vi "MegaAwesome_8_29_12a_JW.vi"() -> ()   [LabVIEW 2011]
uses:
  MegaAwesome_States.ctl
panel:
  out "Folder Index":dbl caption="Length"
  out "Image Preview":T1(plugin-control)
  out "Sat Id-Used":dbl[](array[numeric])
  out "Sat Vg Array-Used":dbl[](array[numeric])
  out "Vg Array-Log-Used":dbl[](array[numeric])
  out "Sat Id-Log-Used":dbl[](array[numeric])
  out "Lin Id-Used":dbl[](array[numeric])
  out "Lin-Vg Array-Used":dbl[](array[numeric])
  out "Lin Vd":dbl
  out "Recorded Prop":T2
  out "Current State":T3
  in  "Main Tab Control":T4(tab)
  in  "Image Folder":path
  out "Image File":path=path "D:/UserData/Desktop/Jeremy/WFU/Research/Programs/VI mods/Image Not Found.png"
  in  "Transfer File":path
  out "Transfer Folder":path
  out "Fabrication Prop":T5
  in  "File Controls":T6
  out "Date Recorded":string="Date Recorded" caption="Measured"
  out "Data Name:":string
  out "Image Name":string
  out "Index":string
  out "Date Created":string caption="Fabricated"
  in  "Comments:":string
  out "Rec: Length":dbl caption="Length" format="%#_3g"
  out "Rec: Width":dbl caption="Width" format="%#_4g"
  out "Rec: Dielectric (d)":dbl caption="Dielectric (d)" format="%#_3g"
  in  "New: Dielectric":dbl
  in  "New: Length":dbl
  in  "New: Width":dbl
  out "Rec: Temp":dbl caption="Sample Temp" format="%.1f"
  in  "New: Temp":dbl format="%.1f"
  in  "Independant Variable":string(combo)="Length (um):"
  out "Image Out":T1(plugin-control)
  in  "Num Pts":dbl=5.0
  in  "Num Pts Log":dbl=5.0 caption="Num Pts"
  out "Recorded Values Cluster":T7
  out "Calculated Values Cluster":T7 caption="Recorded Values Cluster"
  out "Re-Calculated Values Cluster":T7 caption="Recorded Values Cluster"
  in  "Origin Project File":path=path "\\\\acad1\\physics/Jurchescu-group/JW-PD/Group Library/Origin Project Files/DeviceData_8_10_12a_JW.opj"
  in  "No Image File":path=path "\\\\acad1\\physics/Jurchescu-group/JW-PD/Mega Awesome/Image Not Found.png"
  in  "Room Temp":dbl=294.0
  # "Image Location"
  # "Recorded"
  # "Calculated"
  # "Re-Calculated"
  # "Manual"
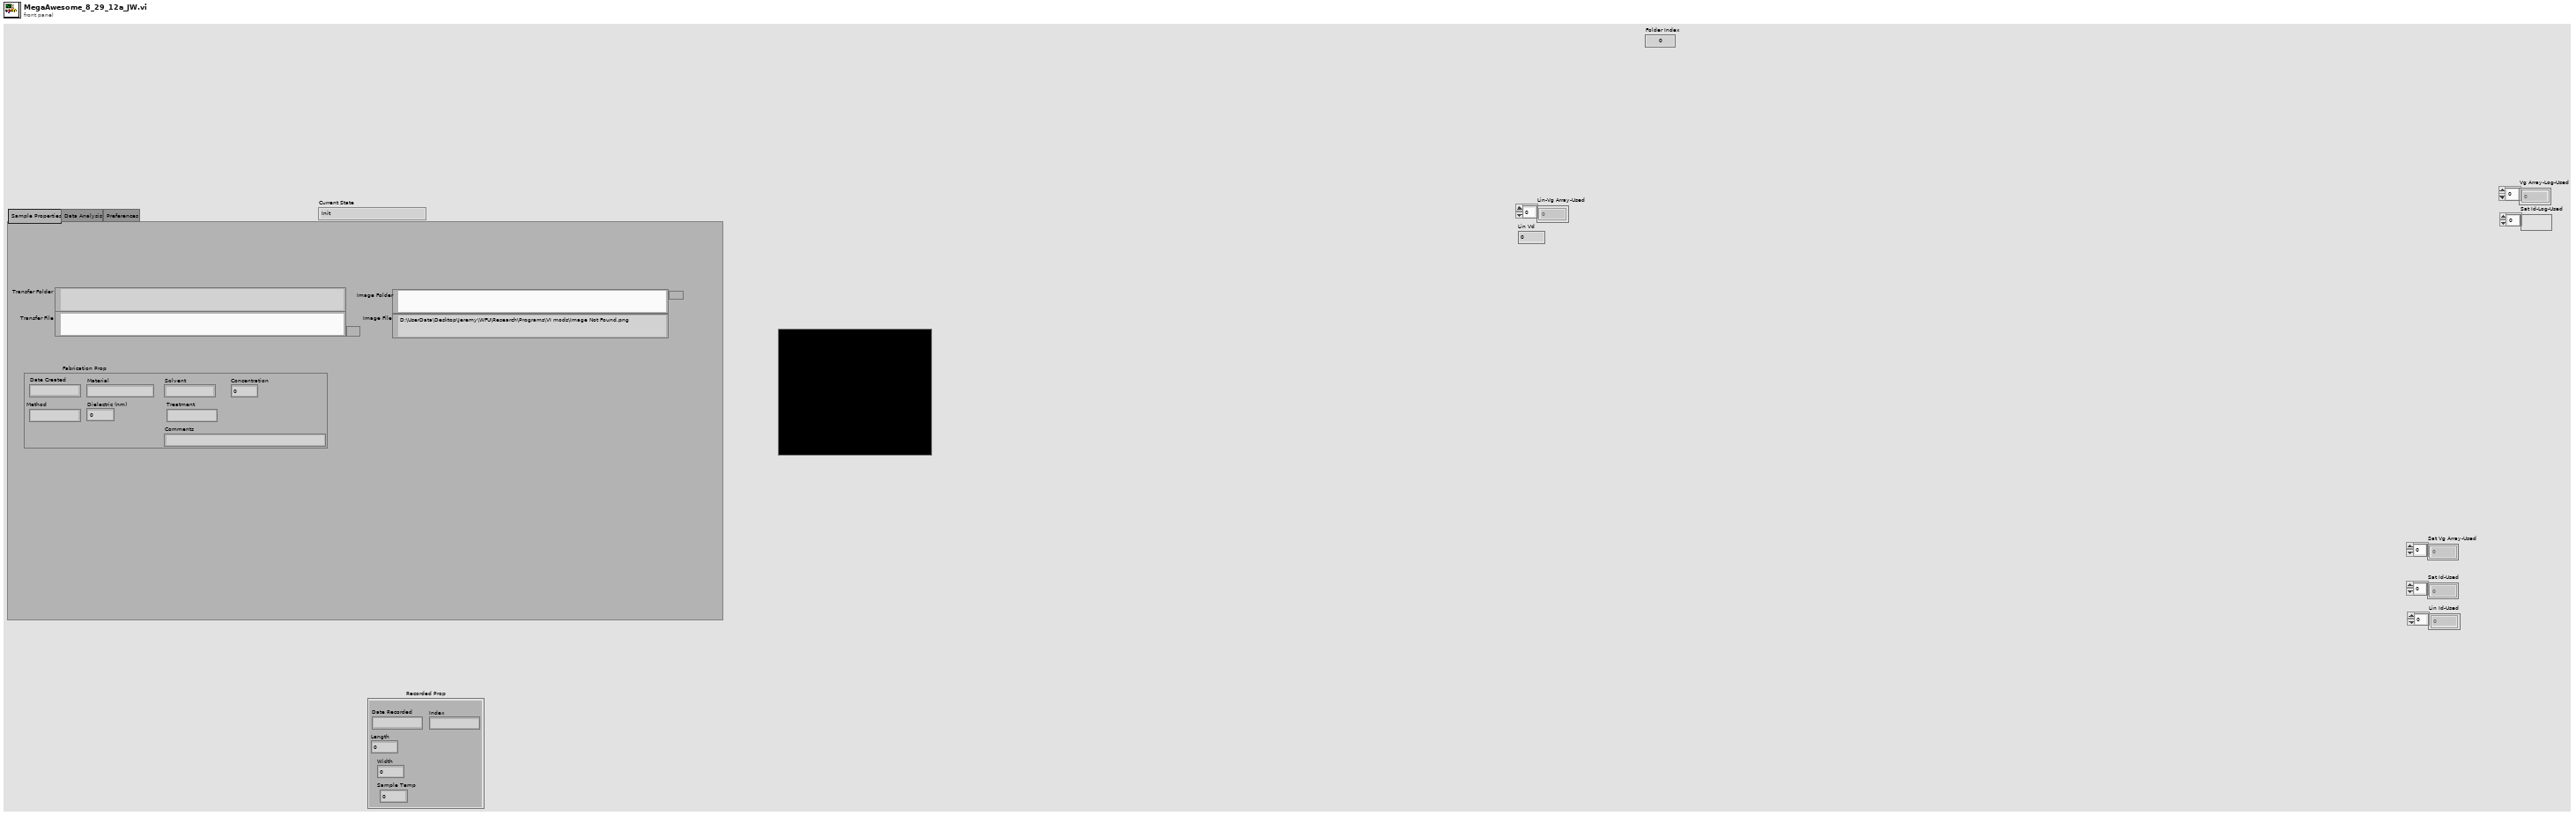
[diagram p1: front panel]
types:
  T1 = typedef "IMAQ Image.ctl" = refnum<image>
  T2 = cluster{"Date Recorded":string, "Index":string, "Length":dbl, "Width":dbl, "Sample Temp":dbl}
  T3 = typedef "MegaAwesome_States.ctl" = enum16{"Init", "File Missing", "No Event", "Read Data", "Calculated Values", "Re-Calculated Values", "Next File", "Previous File", "Discard File", "Save", "Save Lines", "Export", "Exit"}
  T4 = enum32{"Sample Properties", "Data Analysis", "Preferences"}
  T5 = cluster{"Date Created":string, "Material":string, "Solvent":string, "Concentration":dbl, "Method":string, "Dielectric (nm)":dbl, "Treatment":string, "Comments":string}
  T6 = cluster{"Previous File":bool, "Discard ":bool, "Save Lines":bool, "Close":bool, "Next File ":bool, "Save":bool, "Save Next":bool, "Export":bool}
  T7 = cluster{"Mobility-Sat":dbl, "Moblitity-Lin":dbl, "On/Off":dbl, "Off Current":dbl, "Vt-Sat":dbl, "STS":dbl, "Trap Density-VT":dbl, "Trap Density-STS":dbl}
  T8 = cluster{"Mobility-Sat":dbl, "Vt-Sat":dbl, "Mobility-Lin":dbl, "Vt-Lin":dbl, "Off I-Sat":dbl, "On/Off I-Sat":dbl}
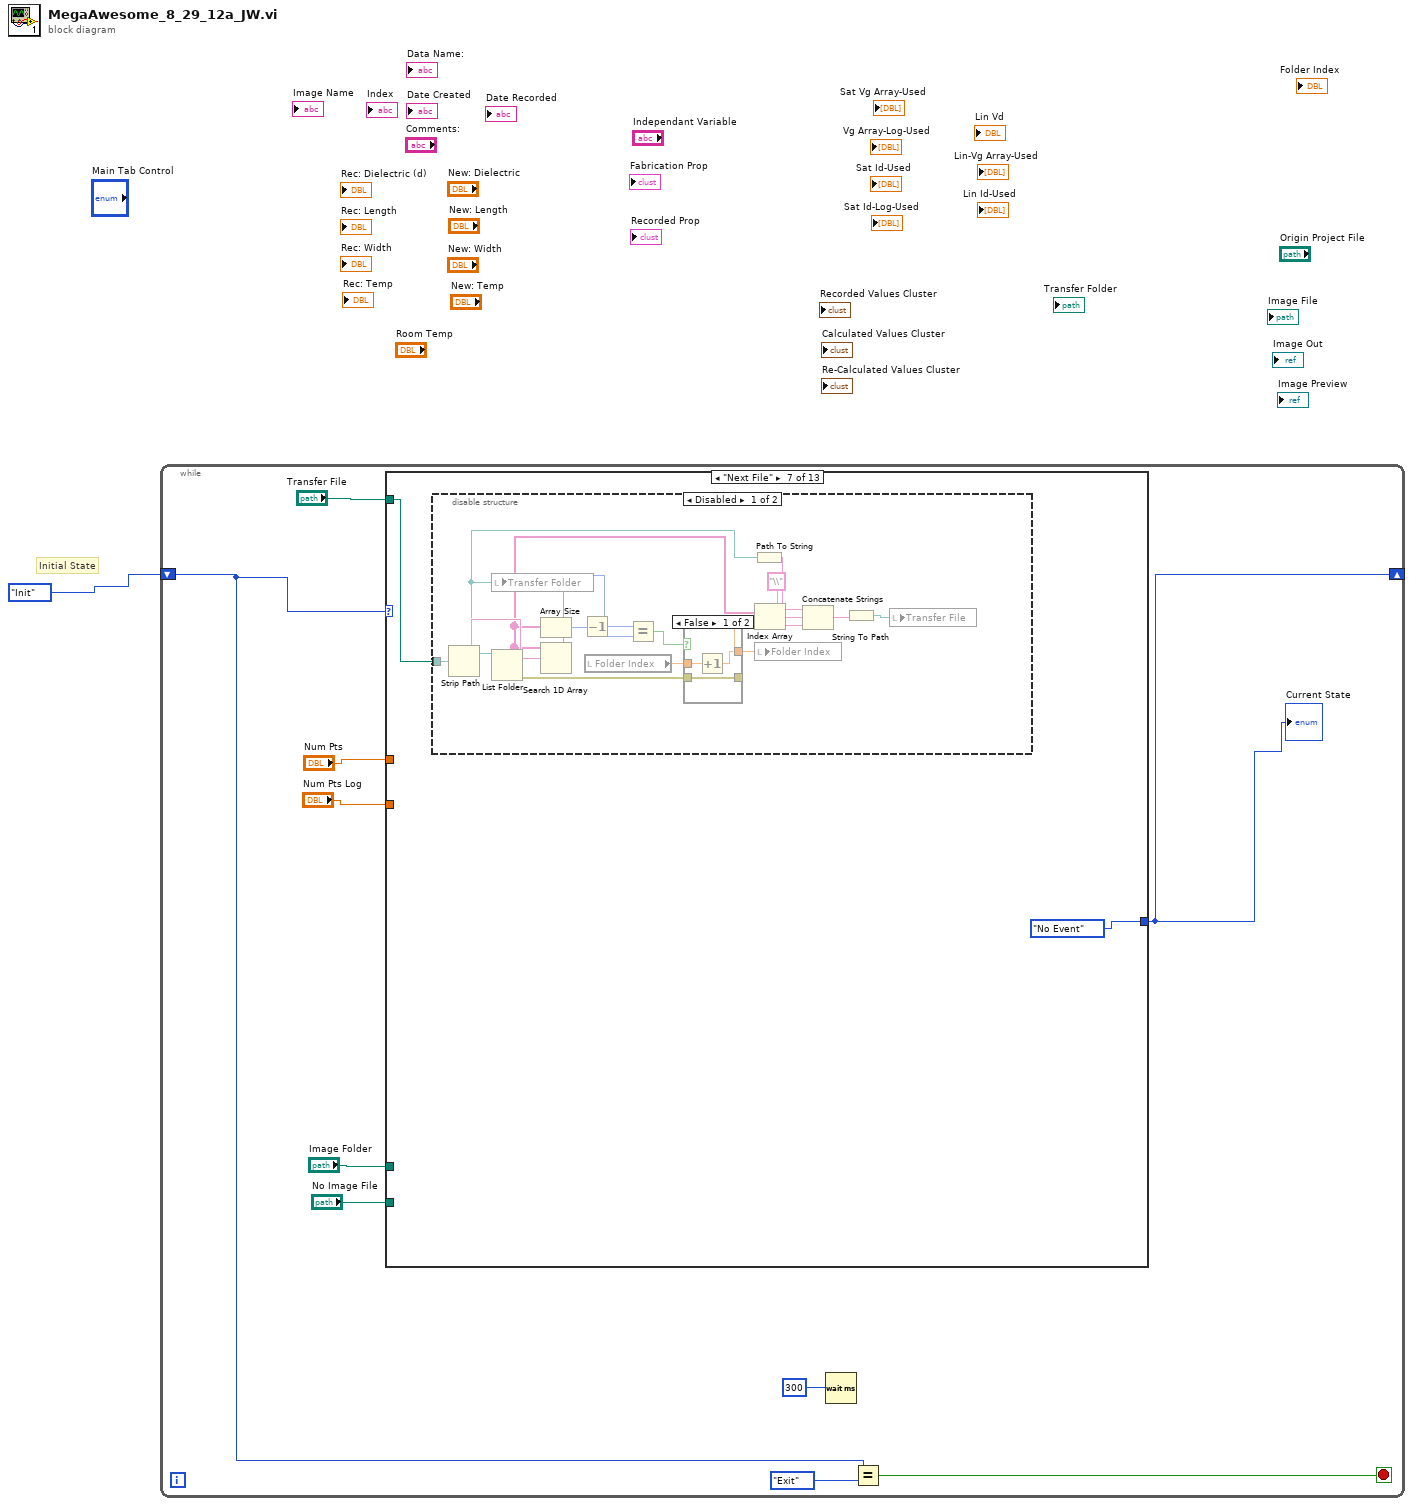
[diagram p0: block diagram]
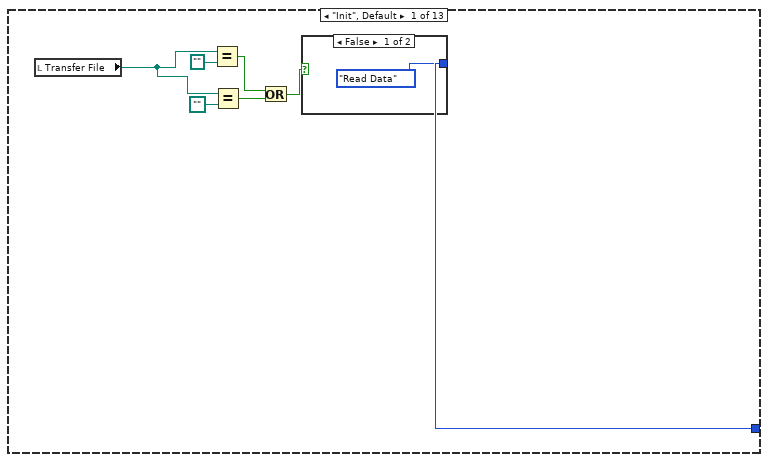
[diagram p2: hidden frame]
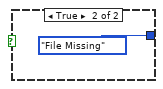
[diagram p3: hidden frame]
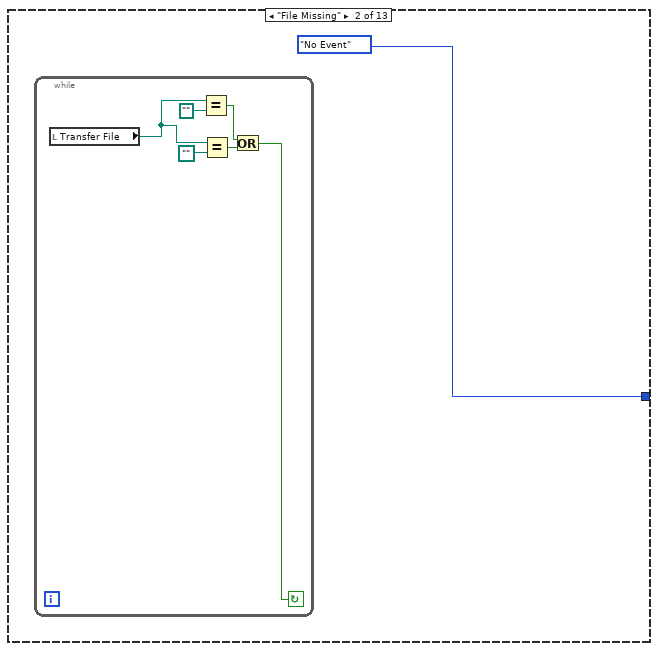
[diagram p4: hidden frame]
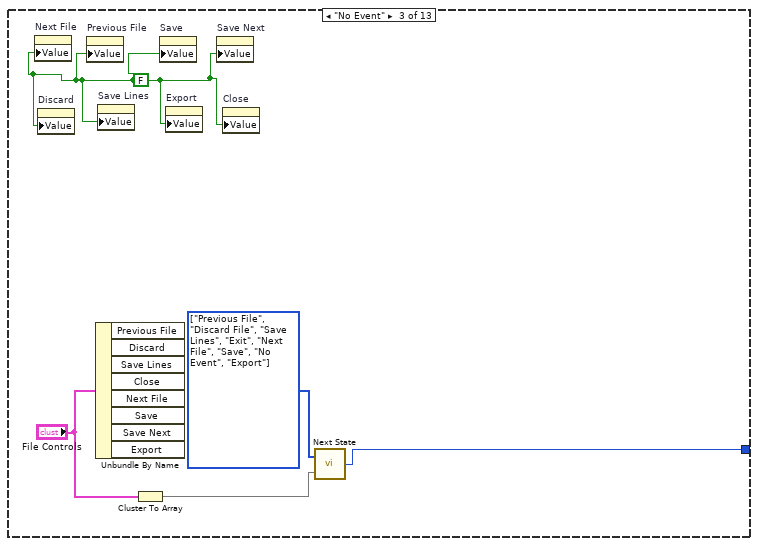
[diagram p5: hidden frame]
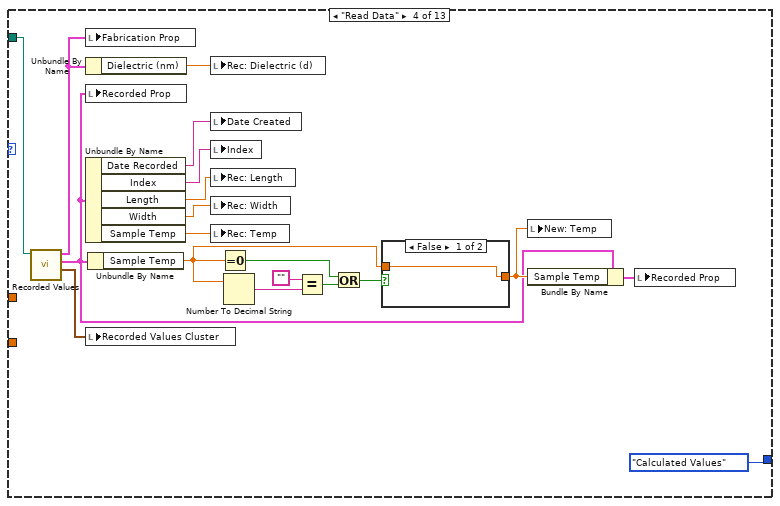
[diagram p6: hidden frame]
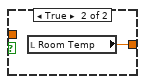
[diagram p7: hidden frame]
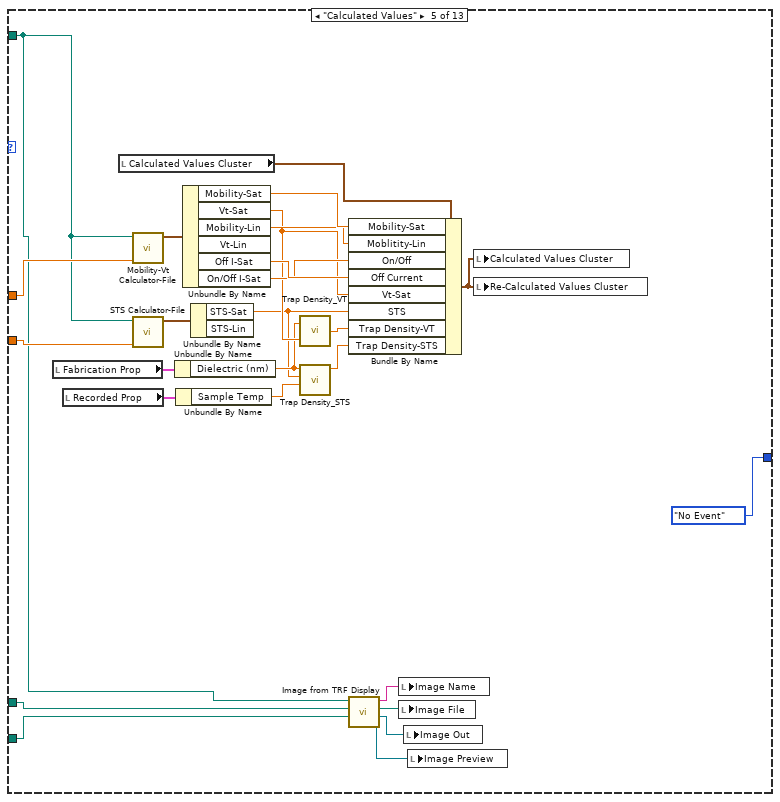
[diagram p8: hidden frame]
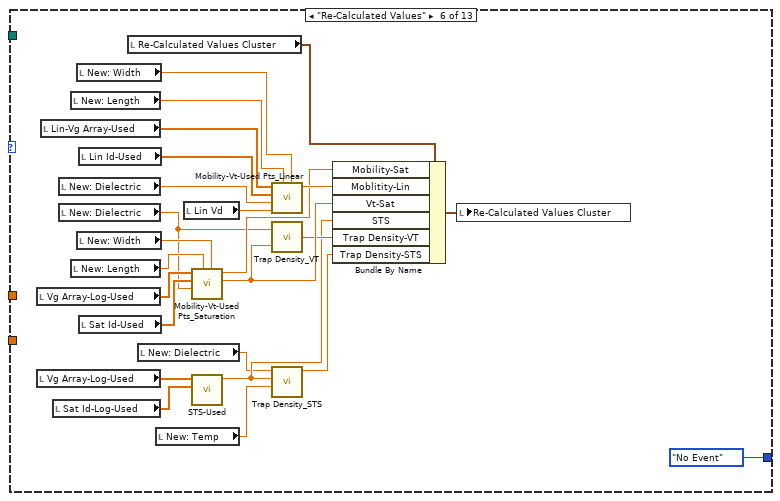
[diagram p9: hidden frame]
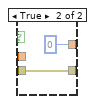
[diagram p10: hidden frame]
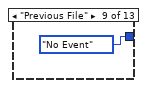
[diagram p13: hidden frame]
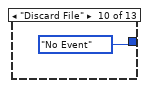
[diagram p14: hidden frame]
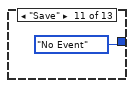
[diagram p15: hidden frame]
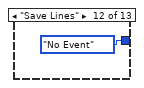
[diagram p16: hidden frame]
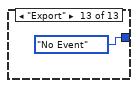
[diagram p17: hidden frame]
diagram:
  # "Initial State"
  n1 = while {
    shift-right: [w7] -> _
    shift-left: MegaAwesome_States."Init" -> [w10]
    stop <- w11 stop-if-true
    n2 = case shown="\"Next File\"" w10 {
      selector: w10 -> [_ _ _ _ _ _ _ w127 _ _ _ _ _]
      tunnel: [w12 MegaAwesome_States."No Event" w30 MegaAwesome_States."Calculated Values" MegaAwesome_States."No Event" MegaAwesome_States."No Event" MegaAwesome_States."No Event" w127 MegaAwesome_States."No Event" MegaAwesome_States."No Event" MegaAwesome_States."No Event" MegaAwesome_States."No Event" MegaAwesome_States."No Event"] -> w7
      tunnel: "Transfer File" -> [_ _ _ w51 w60 _ w105 _ _ _ _ _ _]
      tunnel: "Num Pts" -> [_ _ _ _ w64 _ _ _ _ _ _ _ _]
      tunnel: "Num Pts Log" -> [_ _ _ _ w63 _ _ _ _ _ _ _ _]
      tunnel: "Image Folder" -> [_ _ _ _ w59 _ _ _ _ _ _ _ _]
      tunnel: "No Image File" -> [_ _ _ _ w58 _ _ _ _ _ _ _ _]
      frame "Init", Default {
        n3 = local read "Transfer File"() -> (w13:path)
        n4 = Equal?(x=w13, y=path "") -> (x = y?=w16:bool)
        n5 = Equal?(x=w13, y=path "") -> (x = y?=w15:bool)
        n6 = Or(x=w16, y=w15) -> (x .or. y?=w18:bool)
        n7 = case shown="False" w18 {
          tunnel: [MegaAwesome_States."Read Data" MegaAwesome_States."File Missing"] -> w12
          frame False {
          }
          frame True {
          }
        }
      }
      frame "File Missing" {
        n8 = while {
          stop <- w22 continue-if-true
          n9 = local read "Transfer File"() -> (w23:path)
          n10 = Equal?(x=w23, y=path "") -> (x = y?=w25:bool)
          n11 = Equal?(x=w23, y=path "") -> (x = y?=w26:bool)
          n12 = Or(x=w25, y=w26) -> (x .or. y?=w22:bool)
        }
      }
      frame "No Event" {
        w31 = T3[] [enum."Previous File", enum."Discard File", enum."Save Lines", enum."Exit", enum."Next File", enum."Save", enum."No Event", enum."Export"] items=["Init", "File Missing", "No Event", "Read Data", "Calculated Values", "Re-Calculated Values", "Next File", "Previous File", "Discard File", "Save", "Save Lines", "Export", "Exit"]
        w32 = FALSE
        n13 = property on="Next File" class="Bool (strict)"("Value"=w32) -> ()  [unwired: 2 in, 2 out]
        n14 = property on="Discard" class="Bool (strict)"("Value"=w32) -> ()  [unwired: 2 in, 2 out]
        n15 = property on="Previous File" class="Bool (strict)"("Value"=w32) -> ()  [unwired: 2 in, 2 out]
        n16 = Unbundle By Name("File Controls") -> ()  [unwired: 8 out]
        n17 = property on="Save Lines" class="Bool (strict)"("Value"=w32) -> ()  [unwired: 2 in, 2 out]
        n18 = Cluster To Array(cluster="File Controls") -> (array=w28:bool[])
        n19 = property on="Save" class="Bool (strict)"("Value"=w32) -> ()  [unwired: 2 in, 2 out]
        n20 = property on="Export" class="Bool (strict)"("Value"=w32) -> ()  [unwired: 2 in, 2 out]
        n21 = property on="Save Next" class="Bool (strict)"("Value"=w32) -> ()  [unwired: 2 in, 2 out]
        n22 = property on="Close" class="Bool (strict)"("Value"=w32) -> ()  [unwired: 2 in, 2 out]
        n23 = call "Next State.vi"("Buttons []"=w28, "States []"=w31) -> ("Enum"=w30:T3)
      }
      frame "Read Data" {
        n24 = call "Recorded Values.vi"("Path"=w51) -> ("Recorded Char"=w50:T7, "Recorded Prop"=w40:T2, "Fabrication Prop"=w34:T5)  [unwired: 8 in]
        n25 = local write "Fabrication Prop"(w34) -> ()
        n26 = Unbundle By Name(w34) -> ("Dielectric (nm)"=w33:dbl)
        n27 = local write "Recorded Prop"(w40) -> ()
        n28 = Unbundle By Name(w40) -> ("Date Recorded"=w39:string, "Index"=w37:string, "Length"=w38:dbl, "Width"=w36:dbl, "Sample Temp"=w35:dbl)
        n29 = local write "Recorded Values Cluster"(w50) -> ()
        n30 = Unbundle By Name(w40) -> ("Sample Temp"=w43:dbl)
        n31 = local write "Rec: Dielectric (d)"(w33) -> ()
        n32 = local write "Date Created"(w39) -> ()
        n33 = local write "Index"(w37) -> ()
        n34 = local write "Rec: Length"(w38) -> ()
        n35 = local write "Rec: Width"(w36) -> ()
        n36 = local write "Rec: Temp"(w35) -> ()
        n37 = Equal To 0?(x=w43) -> (x = 0?=w46:bool)
        n38 = Number To Decimal String(number=w43) -> (decimal integer string=w47:string)  [unwired: 1 in]
        n39 = Equal?(x="", y=w47) -> (x = y?=w45:bool)
        n40 = Or(x=w46, y=w45) -> (x .or. y?=w44:bool)
        n41 = case shown="False" w44 {
          tunnel: [w52 w53] -> w41
          tunnel: w43 -> [w52 _]
          frame False {
          }
          frame True {
            n42 = local read "Room Temp"() -> (w53:dbl)
          }
        }
        n43 = local write "New: Temp"(w41) -> ()
        n44 = Bundle By Name(cluster=w40, "Sample Temp"=w41) -> (w42:T2)
        n45 = local write "Recorded Prop"(w42) -> ()
      }
      frame "Calculated Values" {
        n46 = local read "Fabrication Prop"() -> (w69:T5)
        n47 = local read "Recorded Prop"() -> (w62:T2)
        n48 = local read "Calculated Values Cluster"() -> (w79:T7)
        n49 = call "Mobility-Vt Calculator-File.vi"("NumPts"=w64, "Path"=w60) -> ("Output"=w77:T8)  [unwired: 5 in, 4 out]
        n50 = call "STS Calculator-File.vi"("NumPts"=w63, "Path"=w60) -> ("Ouput"=w72:cluster{"STS-Sat":dbl, "STS-Lin":dbl})  [unwired: 5 in, 4 out]
        n51 = Unbundle By Name(w69) -> ("Dielectric (nm)"=w67:dbl)
        n52 = Unbundle By Name(w62) -> ("Sample Temp"=w61:dbl)
        n53 = Unbundle By Name(w77) -> ("Mobility-Sat"=w76:dbl, "Vt-Sat"=w68:dbl, "Mobility-Lin"=w75:dbl, "Off I-Sat"=w74:dbl, "On/Off I-Sat"=w73:dbl)  [unwired: 1 out]
        n54 = Unbundle By Name(w72) -> ("STS-Sat"=w66:dbl)  [unwired: 1 out]
        n55 = call "Trap Density_VT.vi"("VT"=w68, "Dielectric"=w67) -> ("Trap Density-VT"=w71:dbl)
        n56 = call "Trap Density_STS.vi"("Temp (T) [K]"=w61, "S.T.S. (S)"=w66, "Dielectric"=w67) -> ("Trap Density (N)"=w70:dbl)  [unwired: 8 in]
        n57 = Bundle By Name(cluster=w79, "Mobility-Sat"=w76, "Moblitity-Lin"=w75, "On/Off"=w73, "Off Current"=w74, "Vt-Sat"=w68, "STS"=w66, "Trap Density-VT"=w71, "Trap Density-STS"=w70) -> (w78:T7)
        n58 = call "Image from TRF Display.vi"("No Image File"=w58, "Image Folder"=w59, "Transfer File"=w60) -> ("Image Out 2"=w54:T1, "Image Out"=w55:T1, "Image File"=w56:path, "Image Name"=w57:string)  [unwired: 5 in]
        n59 = local write "Image Name"(w57) -> ()
        n60 = local write "Image File"(w56) -> ()
        n61 = local write "Image Out"(w55) -> ()
        n62 = local write "Image Preview"(w54) -> ()
        n63 = local write "Calculated Values Cluster"(w78) -> ()
        n64 = local write "Re-Calculated Values Cluster"(w78) -> ()
      }
      frame "Re-Calculated Values" {
        n65 = local read "Vg Array-Log-Used"() -> (w94:dbl[])
        n66 = local read "Vg Array-Log-Used"() -> (w86:dbl[])
        n67 = local read "Lin-Vg Array-Used"() -> (w101:dbl[])
        n68 = local read "Sat Id-Log-Used"() -> (w85:dbl[])
        n69 = local read "New: Dielectric"() -> (w99:dbl)
        n70 = local read "New: Dielectric"() -> (w83:dbl)
        n71 = local read "New: Length"() -> (w97:dbl)
        n72 = local read "New: Length"() -> (w93:dbl)
        n73 = local read "New: Width"() -> (w96:dbl)
        n74 = local read "New: Width"() -> (w92:dbl)
        n75 = local read "Lin Id-Used"() -> (w100:dbl[])
        n76 = local read "Sat Id-Used"() -> (w91:dbl[])
        n77 = local read "Re-Calculated Values Cluster"() -> (w103:T7)
        n78 = local read "New: Dielectric"() -> (w82:dbl)
        n79 = local read "New: Temp"() -> (w81:dbl)
        n80 = local read "Lin Vd"() -> (w98:dbl)
        n81 = call "Mobility-Vt-Used Pts_Saturation.vi"("Width"=w92, "Length"=w93, "Dielectric (d)"=w83, "Sat Id Used"=w91, "Vg Used"=w94) -> ("Vt"=w89:dbl, "Mobility"=w90:dbl)  [unwired: 4 in, 1 out]
        n82 = call "STS-Used.vi"("Id Used"=w85, "Vg-Used"=w86) -> ("STS"=w84:dbl)  [unwired: 9 in]
        n83 = call "Mobility-Vt-Used Pts_Linear.vi"("Width"=w96, "Length"=w97, "Vd"=w98, "Dielectric (d)"=w99, "Sat Id Used"=w100, "Vg Used"=w101) -> ("Mobility"=w95:dbl)  [unwired: 3 in, 2 out]
        n84 = call "Trap Density_VT.vi"("VT"=w89, "Dielectric"=w83) -> ("Trap Density-VT"=w88:dbl)
        n85 = call "Trap Density_STS.vi"("Temp (T) [K]"=w81, "S.T.S. (S)"=w84, "Dielectric"=w82) -> ("Trap Density (N)"=w80:dbl)  [unwired: 8 in]
        n86 = Bundle By Name(cluster=w103, "Mobility-Sat"=w90, "Moblitity-Lin"=w95, "Vt-Sat"=w89, "STS"=w84, "Trap Density-VT"=w88, "Trap Density-STS"=w80) -> (w102:T7)
        n87 = local write "Re-Calculated Values Cluster"(w102) -> ()
      }
      frame "Next File" {
        n88 = disable-structure shown="Disabled" {
          disable-tunnel: w105 -> [w121 _]
          frame Disabled {
            n89 = Strip Path(path=w121) -> (stripped path=w109:path, name=w120:string)
            n90 = local write "Transfer Folder"(w109) -> ()
            n91 = List Folder(path=w109) -> (folder names=w119:string[], error out=w113:errorcluster)  [unwired: 3 in, 2 out]
            n92 = Array Size(array=w119) -> (size(s)=w118:i32)
            n93 = Search 1D Array(1D array=w119, element=w120) -> (index of element=w116:i32)  [unwired: 1 in]
            n94 = Decrement(x=w118) -> (x-1=w117:i32)
            n95 = local read "Folder Index"() -> (w114:dbl)
            n96 = Equal?(x=w117, y=w116) -> (x = y?=w115:bool)
            n97 = case shown="False" w115 {
              tunnel: w114 -> [w124 _]
              tunnel: [w123 0] -> w112
              tunnel: w113 -> [w122 w125]
              tunnel: [w122 w125] -> _
              frame False {
                n98 = Increment(x=w124) -> (x+1=w123:dbl)
              }
              frame True {
              }
            }
            n99 = Path To String(path=w109) -> (string=w110:string)
            n100 = Index Array(array=w119, index=w112) -> (element=w111:string)
            n101 = local write "Folder Index"(w112) -> ()
            n102 = Concatenate Strings(w110, "\\", w111) -> (w107:string)
            n103 = String To Path(string=w107) -> (path=w106:path)
            n104 = local write "Transfer File"(w106) -> ()
          }
          frame Enabled {
          }
        }
      }
      frame "Exit" {
      }
      frame "Previous File" {
      }
      frame "Discard File" {
      }
      frame "Save" {
      }
      frame "Save Lines" {
      }
      frame "Export" {
      }
    }
    "Current State" <- w7
    n105 = Wait (ms)(milliseconds to wait=300) -> ()  [unwired: 1 out]
    n106 = Equal?(x=w10, y=MegaAwesome_States."Exit") -> (x = y?=w11:bool)
  }
